vi "DisplayName.vi"(1 "State In":T1) -> (0 "Name":string)   [LabVIEW 2010, in "CData Flatten XNode.xnode"]
doc: "This ability is deprecated; prefer GetDisplayName2.\n\nThis ability VI is used to supply LabVIEW with the name of your XNode. This is used as the default value for the label, it is used to mark entries in the error list and the difference list.\n\nDefault behavior: None.\n\nThis ability does not provide UI and OS messages are not handled."
uses:
  CData Flatten XNode.xnode
  State.ctl
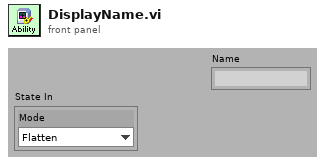
[diagram p1: front panel]
types:
  T1 = typedef "CData Flatten XNode.xnode/State.ctl" = cluster{"Mode":enum16{"Flatten", "Unflatten"}}
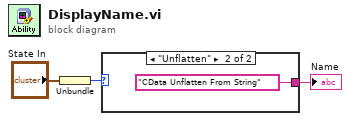
[diagram p0: block diagram]
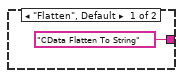
[diagram p2: hidden frame]
diagram:
  n1 = Unbundle("State In") -> ("Mode"=w2:enum16{"Flatten", "Unflatten"})
  n2 = case shown="\"Unflatten\"" w2 {
    tunnel: ["CData Flatten To String" "CData Unflatten From String"] -> w1
    frame "Flatten", Default {
    }
    frame "Unflatten" {
    }
  }
  "Name" <- w1
